vi "DifferentialPositionDutyCycle Setter.vi"(0 "LimitReverseMotion":bool, 1 "EnableFOC":bool=TRUE, 2 "DifferentialSlot":i32=1, 3 "Update Frequency (Hz)":dbl=100.0, 5 "StopSendingOtherRequests":bool=TRUE, 7 "TargetPosition":dbl, 9 "DifferentialPosition":dbl, 12 "TargetSlot":i32, 13 "OverrideBrakeDurNeutral":bool) -> (4 "DeviceReference Out":T1)   [LabVIEW 2023]
doc: "Request PID to target position with a differential position setpoint.\nThis control mode will set the motor's position setpoint to the position specified by the user. It will also set the motor's differential position setpoint to the specified position."
uses:
  Users/Cory/Documents/PhoenixPro-LabVIEW-Generation/controls/DeviceReference.ctl
panel:
  in  "LimitForwardMotion":bool
  in  "DeviceReference":T1
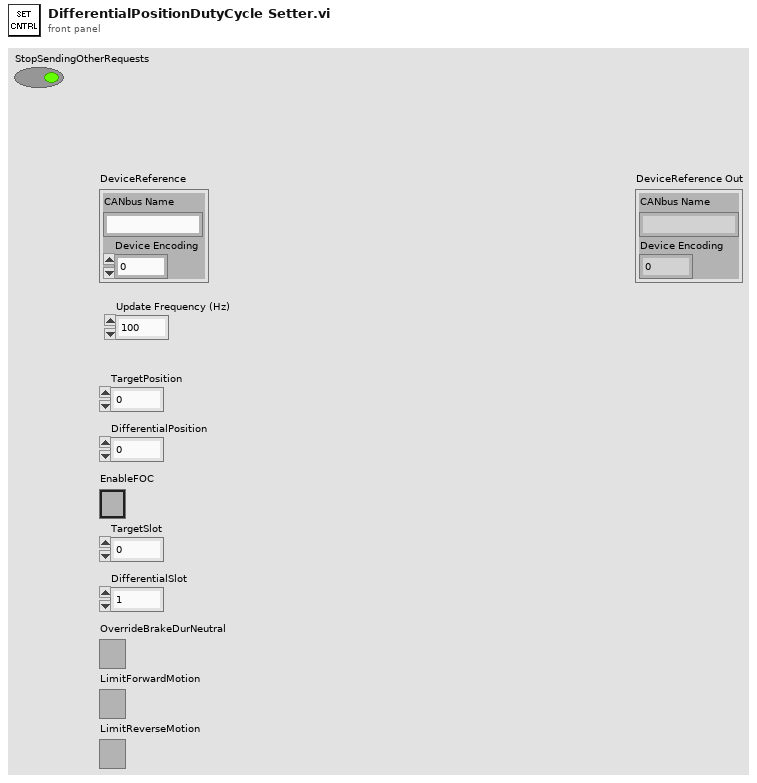
[diagram p1: front panel]
types:
  T1 = typedef "DeviceReference.ctl" = cluster{"CANbus Name":string, "Device Encoding":u32}
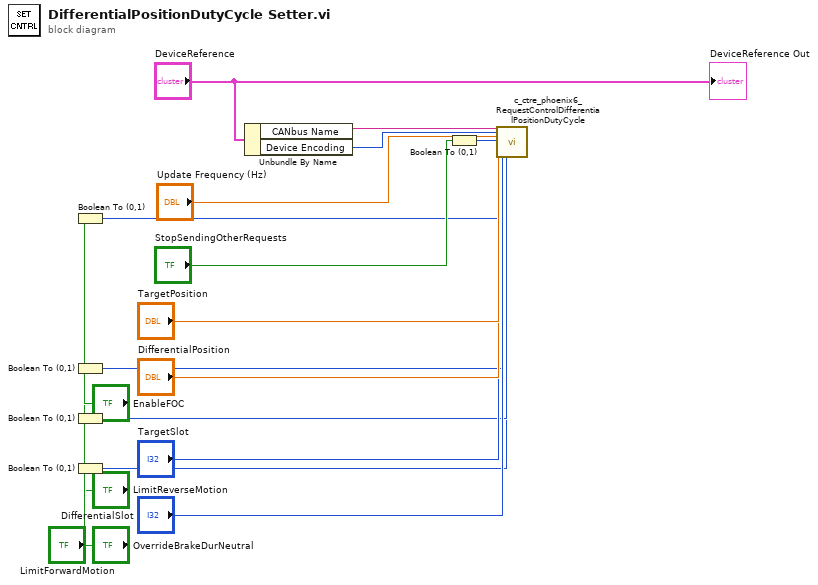
[diagram p0: block diagram]
diagram:
  n1 = Boolean To (0,1)(Boolean="EnableFOC") -> (0, 1=w9:i16)
  n2 = Boolean To (0,1)(Boolean="OverrideBrakeDurNeutral") -> (0, 1=w5:i16)
  n3 = Boolean To (0,1)(Boolean="LimitForwardMotion") -> (0, 1=w3:i16)
  n4 = Boolean To (0,1)(Boolean="LimitReverseMotion") -> (0, 1=w1:i16)
  n5 = Unbundle By Name("DeviceReference") -> ("CANbus Name"=w17:string, "Device Encoding"=w16:u32)
  n6 = Boolean To (0,1)(Boolean="StopSendingOtherRequests") -> (0, 1=w13:i16)
  n7 = call <vilib>:"c_ctre_phoenix6_RequestControlDifferentialPositionDutyCycle.vi"("String 2"=w17, "Numeric 2"=w16, "Numeric 3"="Update Frequency (Hz)", "Numeric 4"=w13, "Numeric 5"="TargetPosition", "Numeric 6"="DifferentialPosition", "Numeric 7"=w9, "Numeric 8"="TargetSlot", "Numeric 9"="DifferentialSlot", "Numeric 10"=w5, "Numeric 11"=w3, "Numeric 12"=w1) -> ()  [unwired: 14 in, 2 out]
  "DeviceReference Out" <- "DeviceReference"
